vi "runscenario zip up files.vi"(8 "error in (no error)":errorcluster, 9 "Filenames to Zip (empty)":string[](array[string]), 10 "Path to Files (empty)":path, 11 "Zip filename (\"\")":string) -> (0 "error out":errorcluster, 3 "Content":string)   [LabVIEW 2011]
uses:
  OpenG.LIB/file/file.llb/File Exists - Scalar__ogtk.vi
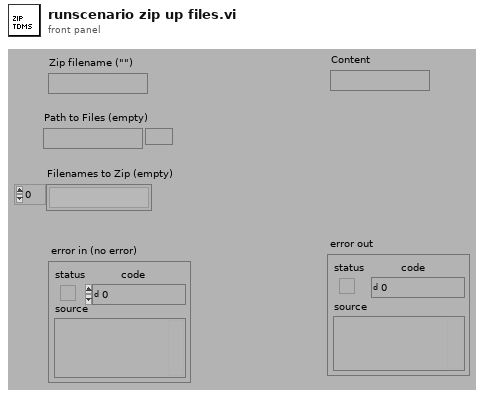
[diagram p1: front panel]
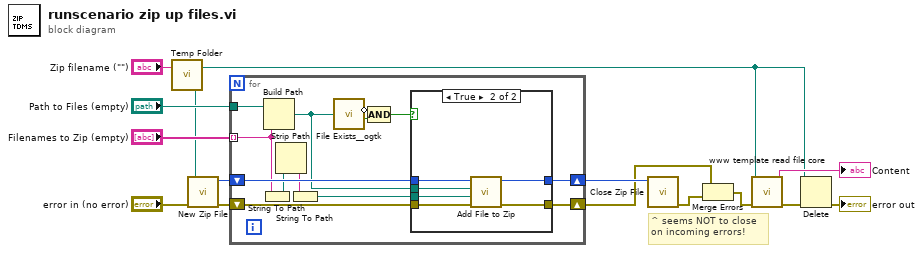
[diagram p0: block diagram]
diagram:
  # "^ seems NOT to close\non incoming errors!"
  n1 = call "Temp Folder.vi"("Relative Path (\"\")"="Zip filename (\"\")") -> ("Temp Folder"=w2:path)  [unwired: 2 in]
  n2 = call <vilib>:"New Zip File.vi"("error in (no error)"="error in (no error)", "target"=w2) -> ("error out"=w13:errorcluster, "zip file out"=w12:i64)  [unwired: 1 in, 3 out]
  n3 = for {
    tunnel: "Path to Files (empty)" -> [w27]
    tunnel: "Filenames to Zip (empty)" -> [w22] mode=indexing
    shift-right: [w25] -> w9
    shift-left: w13 -> [w26]
    shift-right: [w24] -> w11
    shift-left: w12 -> [w23]
    n4 = String To Path(string=w22) -> (path=w17:path)
    n5 = Build Path(base path=w27, name or relative path=w22) -> (appended path=w21:path)
    n6 = Strip Path(path=w17) -> (name=w16:string)  [unwired: 1 out]
    n7 = String To Path(string=w16) -> (path=w15:path)
    n8 = call-poly "File Exists__ogtk.vi"("file path"=w21) -> ("is directory"=w19:bool, "exists"=w20:bool)  [unwired: 6 in]
    n9 = Compound Arithmetic op=AND(invert w19, w20) -> (w18:bool)
    n10 = case shown="True" w18 {
      tunnel: w26 -> [w28 w35]
      tunnel: [w28 w34] -> w25
      tunnel: [w29 w33] -> w24
      tunnel: w23 -> [w29 w32]
      tunnel: w15 -> [_ w31]
      tunnel: w21 -> [_ w30]
      frame False {
      }
      frame True {
        n11 = call <vilib>:"Add File to Zip.vi"("error in (no error)"=w35, "destination path in zip"=w31, "source file path"=w30, "zip file in"=w32) -> ("error out"=w34:errorcluster, "zip file out"=w33:i64)  [unwired: 6 out]
      }
    }
  }
  n12 = call <vilib>:"Close Zip File.vi"("zip file in"=w11) -> ("error out"=w8:errorcluster)  [unwired: 2 in, 4 out]
  n13 = Merge Errors(w9, w8) -> (w10:errorcluster)
  n14 = call "www template read file core.vi"("error in (no error)"=w10, "Path"=w2) -> ("error out"=w14:errorcluster, "File Content"=→"Content":string)  [unwired: 8 out]
  n15 = Delete(path (use dialog)=w2, error in=w14) -> (error out=→"error out":errorcluster)  [unwired: 5 out]
